vi "hms_to_s.vi"(1 "s":i32 min=0 max=59 step=1, 2 "m":i32 min=0 max=59 step=1, 3 "h":i32 min=0 max=23 step=1) -> (0 "result":i32)   [LabVIEW 2019]
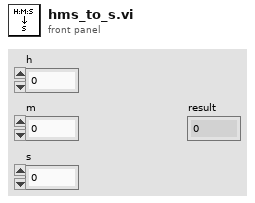
[diagram p1: front panel]
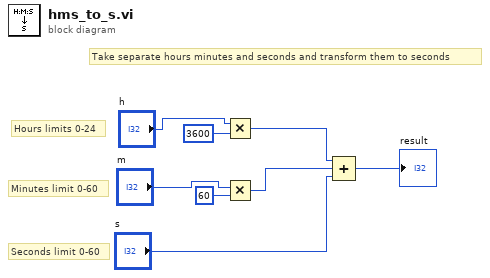
[diagram p0: block diagram]
diagram:
  # "Seconds limit 0-60"
  # "Minutes limit 0-60"
  # "Hours limits 0-24"
  # "Take separate hours minutes and seconds and transform them to seconds"
  n1 = Multiply(x="h", y=3600) -> (x*y=w5:i32)
  n2 = Multiply(x="m", y=60) -> (x*y=w6:i32)
  n3 = Compound Arithmetic op=ADD(w5, w6, "s") -> (→"result":i32)
